vi "HEWH RLT PRAT.vi"() -> ()   [LabVIEW 2016] (continued)
      n10 = local write "Outlet Valve A"(w132) -> ()
      n11 = local write "Outlet Valve B"(w132) -> ()
      n12 = local write "Outlet Valve C"(w132) -> ()
      n13 = local write "Outlet Valve D"(w132) -> ()
      n14 = local write "Draw Complete"(w135) -> ()
      n15 = local write "DAQ Finished"(w135) -> ()
      n16 = local write "Init Complete"(w134) -> ()
      n17 = local write "Finish"(w134) -> ()
      n18 = local write "Alarm A"(w134) -> ()
      n19 = local write "Alarm B"(w134) -> ()
      n20 = local write "Start Draw Loop"(w134) -> ()
      n21 = local write "Alarm C"(w134) -> ()
      n22 = local write "Start/Pause test"(w134) -> ()
      n23 = local write "Alarm D"(w134) -> ()
      n24 = local write "Use Agilent?"(w134) -> ()
      n25 = local write "Disable Station 1"(w137) -> ()
      n26 = local write "Disable Station 2"(w137) -> ()
      n27 = local write "Disable Station 3"(w137) -> ()
      n28 = local write "Disable Station 4"(w137) -> ()
      n29 = local write "Shutdown"("" ("Shutdown")) -> ()
      n30 = disable-structure shown="Disabled" {
        frame Disabled {
          n31 = call "UTILITY Startup and Initialize.vi"() -> ()  [unwired: 24 in, 4 out]
        }
        frame Enabled {
        }
      }
    }
  }
  n32 = call "HEWH Power Notifier.vi"("Status"=w99, "error in (no error)"=w105, "Set Status"=w98, "name (unnamed)"="PowerA") -> ("error out"=w104:errorcluster)  [unwired: 6 in, 1 out]
  n33 = call "HEWH Power Notifier.vi"("Status"=w99, "error in (no error)"=w104, "Set Status"=w98, "name (unnamed)"="PowerB") -> ("error out"=w102:errorcluster)  [unwired: 6 in, 1 out]
  n34 = call "HEWH Power Notifier.vi"("Status"=w99, "error in (no error)"=w102, "Set Status"=w98, "name (unnamed)"="PowerC") -> ("error out"=w101:errorcluster)  [unwired: 6 in, 1 out]
  n35 = call "HEWH Power Notifier.vi"("Status"=w99, "error in (no error)"=w101, "Set Status"=w98, "name (unnamed)"="PowerD") -> ("error out"=w55:errorcluster)  [unwired: 6 in, 1 out]
  n36 = Current VI's Path() -> (path=w58:path)
  n37 = call "UTILITY This VIs Path.vi"("path"=w58, "error in (no error)"=w55) -> ("Folder Path"=w53:path, "FileVersionInfo Out"=w59:T5, "error out"=w54:errorcluster)  [unwired: 7 in, 4 out]
  n38 = Unbundle By Name(w59) -> ("FileVersion"=→"File  Version":string)
  n39 = call "HEWH Read Settings.vi"("Tool Base Path"=w53, "Error In"=w54) -> ("K-Factor Intellifaucet"=→"K-Factor Intellifaucet":dbl, "Power Analyzer"=→"Power Analyzer":T11, "Station"=→"Station":string, "LV Program"=w64:T24, "Error Out"=w65:errorcluster)  [unwired: 13 in]
  "LV Program" <- w64
  n40 = case shown="\"HEWH\", Default" w64 {
    tunnel: [Save_File_RLT_Station_Type."Single Station" ("RLT Station Type") Save_File_RLT_Station_Type."Four Stations" ("RLT Station Type")] -> w52
    frame "HEWH", Default {
      w140 = FALSE ("New File Per CycA")
      n41 = local write "New File Per CycA"(w140) -> ()
      n42 = local write "New File Per CycB"(w140) -> ()
      n43 = local write "New File Per CycC"(w140) -> ()
      n44 = local write "New File Per CycD"(w140) -> ()
    }
    frame "PRAT", "HEWH RLT" {
      w142 = TRUE ("New File Per CycA")
      n45 = local write "New File Per CycA"(w142) -> ()
      n46 = local write "New File Per CycB"(w142) -> ()
      n47 = local write "New File Per CycC"(w142) -> ()
      n48 = local write "New File Per CycD"(w142) -> ()
    }
  }
  n49 = call <vilib>:"Obtain Semaphore Reference.vi"("error in (no error)"=w65, "name (unnamed)"="MW100") -> ("error out"=w96:errorcluster, "semaphore"=w78:T56)  [unwired: 3 in, 1 out]
  n50 = Create User Event(user event datatype=w110, error in=w96) -> (user event=w24:refnum<user-event>, error out=w108:errorcluster)
  n51 = Create User Event(user event datatype=w109, error in=w108) -> (user event=w107:refnum<user-event>, error out=w82:errorcluster)
  n52 = Create User Event(user event datatype=w83, error in=w82) -> (user event=w23:refnum<user-event>, error out=w1:errorcluster)
  n53 = Create User Event(user event datatype=w68, error in=w1) -> (user event=w67:refnum<user-event>, error out=w63:errorcluster)
  n54 = Obtain Queue(name (unnamed)="Start Draw", element data type=T54 {"Start Draw"=FALSE, "Station ID"=enum."A", "Station Draw Info"={"Sequence #"=0.0, "Cycles"=0, "Mode Setting"="", "Flow Rate (GPM)"=0.0, "Temperature (F)"=0.0, "Reset Timer"=FALSE, "Use Temp Decline Method"=FALSE, "Terminate Condition"=enum."C1-Terminate Draw @ Gallon Mark", "Condition Value #1"=0.0, "UE"=FALSE, "LE"=FALSE, "Comp"=FALSE, "Fan"=FALSE, "Test End Time (Sec)"=0.0, "Purge Until Cutout"=FALSE, "Start Conditions"=enum."Heat Source Cutout", "Condition Value #2"=0.0, "Remove Power"=FALSE, "Time"=0.0, "Check Special Cond."=enum."SC2-Check Heat Source (On-C2/Off-C1)", "Condition#"=enum."C1", "Draw Flags"=enum."N/A", "Data Processing Delay (FHD 15sec, UEF 5 Sec)"=0.0, "Test Complete"=FALSE}, "Send Condition"=enum."N/A"}, error in (no error)=w63) -> (queue out=w116:refnum<queue>, error out=w3:errorcluster)  [unwired: 2 in, 1 out]
  n55 = call "UTILITY String Notifier.vi"("Status"=UTILITY_Notifier."Set", "error in (no error)"=w3, "Set Status"="", "name (unnamed)"="TimerA") -> ("error out"=w6:errorcluster)  [unwired: 6 in, 1 out]
  n56 = call "UTILITY String Notifier.vi"("Status"=UTILITY_Notifier."Set", "error in (no error)"=w6, "Set Status"="", "name (unnamed)"="TimerB") -> ("error out"=w5:errorcluster)  [unwired: 6 in, 1 out]
  n57 = call "UTILITY String Notifier.vi"("Status"=UTILITY_Notifier."Set", "error in (no error)"=w5, "Set Status"="", "name (unnamed)"="TimerC") -> ("error out"=w4:errorcluster)  [unwired: 6 in, 1 out]
  n58 = call "UTILITY String Notifier.vi"("Status"=UTILITY_Notifier."Set", "error in (no error)"=w4, "Set Status"="", "name (unnamed)"="TimerD") -> ("error out"=w2:errorcluster)  [unwired: 6 in, 1 out]
  n59 = call "UTILITY String Notifier.vi"("Status"=UTILITY_Notifier."Set", "error in (no error)"=w2, "Set Status"="", "name (unnamed)"="Message") -> ("error out"=w92:errorcluster)  [unwired: 6 in, 1 out]
  n60 = register-events(w107, w23) -> (reference out=w86:refnum<event-registration>)  [unwired: 2 in, 1 out]
  n61 = call "UTILITY Boolean Notifier.vi"("Status"=UTILITY_Notifier."Set", "error in (no error)"=w92, "Set Status"=FALSE, "name (unnamed)"="Stop Custom Draw") -> ("error out"=w74:errorcluster)  [unwired: 6 in, 1 out]
  n62 = call "HEWH Draw Flag.vi"("Station ID"=Station_ID_Selector."Global", "Status"=UTILITY_Notifier."Set", "Error In"=w74) -> ("Error Out"=w73:errorcluster)  [unwired: 8 in, 4 out]
  n63 = Bundle By Name(cluster="File Locations In", "General Setup Paths.Tool Base Path"=w53) -> (w56:T2)
  n64 = call "HEWH Cut Out Flag.vi"("Error In"=w73) -> ("Error Out"=w69:errorcluster)  [unwired: 10 in]
  n65 = call "UTILITY Boolean Notifier.vi"("Status"=UTILITY_Notifier."Set", "error in (no error)"=w69, "Set Status"=FALSE, "name (unnamed)"="Use Last Start Condition") -> ("error out"=w29:errorcluster)  [unwired: 6 in, 1 out]
  n66 = call "HEWH GEA Notifier.vi"("Status"=UTILITY_Notifier."Set", "error in (no error)"=w29, "name (unnamed)"="GEA_A") -> ("error out"=w28:errorcluster)  [unwired: 7 in, 1 out]
  n67 = call "HEWH GEA Notifier.vi"("Status"=UTILITY_Notifier."Set", "error in (no error)"=w28, "name (unnamed)"="GEA_B") -> ("error out"=w27:errorcluster)  [unwired: 7 in, 1 out]
  n68 = call "HEWH GEA Notifier.vi"("Status"=UTILITY_Notifier."Set", "error in (no error)"=w27, "name (unnamed)"="GEA_C") -> ("error out"=w26:errorcluster)  [unwired: 7 in, 1 out]
  n69 = call "HEWH GEA Notifier.vi"("Status"=UTILITY_Notifier."Set", "error in (no error)"=w26, "name (unnamed)"="GEA_D") -> ("error out"=w25:errorcluster)  [unwired: 7 in, 1 out]
  n70 = case shown="\"Single Station\", Default" w52 {
    tunnel: [w145 w156] -> w50
    tunnel: [w145 w155] -> w49
    tunnel: [w145 w154] -> w48
    tunnel: [w146 w153] -> w46
    tunnel: [w146 w152] -> w62
    tunnel: [w146 w151] -> w61
    tunnel: w56 -> [_ w150]
    tunnel: [w144 w149] -> w21
    tunnel: [w144 w148] -> w20
    tunnel: [w144 w147] -> w19
    frame "Single Station", Default {
      w144 = T2 {"General Setup Paths"={"Calibration File Path"=path "", "DOE Capacity Path"=path "", "Data Folder Path"=path "", "RLT Backup Data Path"=path "", "Tool Base Path"=path "", "General Startup Config Path"=path "", "File Save Previous Run Path"=path "", "File Save Configuration Data Path"=path ""}, "Data File Paths"={"Data File Path"=path "", "Debug File Path"=path "", "Bus Log Path"=path "", "Current"=path "", "Summary"=path ""}, "New Summary Created"=FALSE, "Check Location Interval (Second)"=0} ("File Locations Out")
      w145 = T28 {"Appliance Details"={"FileVersionInfo"={"FileVersion"="", "ProductName"="", "InternalName"="", "CompanyName"="", "LegalCopyright"="", "FileDescription"=""}, "Dishwasher Info"={"Open Cup Weight (gm):"=0.0, "Auto Cup Weight (gm):"=0.0, "Detergent-Dish:"="", "Inlet Temperature-Dish:"="", "Cycle Mode-Dish:"="", "Unit Control-Dish:"="", "Manufacturer-Dish:"=""}, "Washer Info"={"Hot Water Temperature (Fahrenheit):"="", "Cold Water Temperature (Fahrenheit):"="", "Capacity (cu.ft):"=0.0, "Initial Cloth Weight:"=0.0, "Cloth Lot:"=0, "Model Family:"="", "Program Name:"="", "Cycle Selection:"="", "Wash Temperature:"="", "Rinse Temperature:"="", "Load Size:"=""}, "File Name Output Array"=[], "Calibration Output Array"=[], "Appliance Common"={"Engineer:"="", "Model Number:"="", "Serial Number:"="", "Comments:"="", "Station ID:"="", "Technician:"="", "TR Number:"="", "Lab ID:"="", "Voltage:"="", "Water Pressure (PSI):"="", "Test Date:"="", "Computer Name:"="", "IP Address:"="", "Ambient RH:"="", "Frequency:"="", "Build:"="", "Filename:"="", "Test Type:"="", "Load Run #:"=0, "Ambient Temperature (F):"="", "File Path:"=path "", "Cycles Per Year"=60}, "Water Heater"={"Heating Mode:"=""}, "Dryer"={"Heat Setting:"="", "Washer Water Temperature (60 ± 5°F):"=60, "Water Hardness (PPM):"=17, "Dryness Setting:"="", "Dryer Type:"="", "Exhaust:"="", "Drying Cycle:"="", "Load Type:"="", "Nominal Load Weight"="", "Dryer Initial IMC Data"={"Measured IMC (lbs)"=7.0, "Actual Initial RMC (%)"=7.0, "RMC (Desired %)"=100.0, "Bone Dry Wt(lbs)"=7.0, "Tolerance(%)"=5.0, "Actual Final RMC (%)"=0.0, "CEF (lbf/kWh)"=0.0, "Minimum Weight (lbf)"=0.0, "Average Weight (lbf)"=0.0, "Maximum Weight (lbf)"=0.0, "Measured IMC In Range?"=FALSE, "Moisture Reduction Factor"=55.5, "Field Use Factor"=1.04, "Empty Dryer Cold Weigth"=0.0, "Energy Standard"=enum."D2-Automatic Dryer", "Weight Cloth (lbs)"=0.0, "Relative Moisture Content (%)"=0.0, "Relative Moisture Content - Avg (%)"=0.0}}}, "Display Data (RLT)"={"Status Color"=0, "Serial Number Display"="", "Cycle Count Display"=0, "Station Label Display"="", "Current Run Start Time Display"=0.0, "Board ID Display"="", "RPM Display"=0, "Current Display"=0.0, "Current Path Display"=path "", "Saving Display"=FALSE, "Unit Type Display"=enum."", "Total Time On Display"=0.0, "UI Button"=FALSE}} ("Main Washer Display Out")
      w146 = T57 {"GEA Diagnostic Data - Washer"={"Speed (RPM)"=0, "Load Size"=0, "Temperature"=0, "Water Pressure"=0.0, "Detergent"=0, "Fabric Softener"=0, "Tub Direction"="", "Detergent Valve"=FALSE, "Fabric Softener Valve"=FALSE, "Recirculating Pump"=FALSE, "Drain Valve"=FALSE, "Hot Valve"=FALSE, "Cold Valve"=FALSE, "Lid Closed Status"="", "Lid Lock Status"="", "Error Count"=0, "IGBT Temperature (Deg C)"=0, "Motor Speed"=0, "Latched OOB"=0, "Raw OOB"=0, "Plaster Status"=0, "Inverter Power (W)"=0, "Target Speed(BRPM)"=0, "Latched Agitate Motor Temp (Deg C)"=0, "Current Motor Temp (Deg C)"=0, "Profiler Status"="", "Current Inverter Action"="", "Error Codes"="", "Lid Locked"=FALSE, "Lid Closed"=FALSE, "9E Diagnostic Data"={"Total Cycle Time (Min)"=0, "Total Cycle Count (Current)"=0, "Total Error Count"=0, "Machine Error History"=0, "Washer UI History"=0, "Inverter Error History"=0, "Cycle Storage Limit"=0, "Error Storage Limit"=0, "Cycle Pages Supported"=0, "Error Pages Supported"=0, "Inverter Reset Count"=0}, "9F Diagnostic Data"={"Cycle Buffer Index"="", "Page Number"="", "Total Cycle Count"=0, "Delay Start Time"=0, "Stain Selected"="", "Selected Cycle"=0, "eWash"="", "Soil Level"="", "Temperature"="", "Overnight Ready"="", "Spin Setting"="", "Control Lock Status"="", "Stain Remover"="", "Steam Assist"="", "My Cycle"="", "PreWash"="", "Debug Log Enabled"="", "Rinse"="", "Signal Level"="", "PreSoak"=""}}, "Software Version"={"Critical Major SW Version"="", "Critical Minor SW Version"="", "Major SW Version"="", "Minor SW Version"="", "Parametric Data Ver. Major"="", "Parametric Data Ver. Minor"="", "Diagnostics Data Ver. Major"="", "Diagnostics Data Ver. Minor"="", "Current Personality Setting"=""}, "Debug Search Parameters"={"Pause"=["MchStdby", "MchPz", "MchIdl", "Machine Standby", "Machine Pause", "Machine Idle"], "Run"=["MchRn", "Machine Run", "Resume Process"], "EOC"=["EOC"], "Error Codes"=["Error1", "try", "rty", "inverr"]}, "Message Count"=0, "Number of Messages"=0, "Partial Message String"="", "Full Message to Save"="", "Board ID"="", "Board Index"=0, "Source Address"=0, "Destination Address"=0, "Data to send"=[], "ReceivedData"=[], "Debug/GEA Data"=[], "Command"=0, "GEA2 Reference Out"=refnum, "GEA2 Event Registration"=refnum, "Bus Data"="", "GEA Data"=[], "Network Variable Location"=0, "Water Heater GEA2 Data"={"GEA2 Label Array"=[], "PID_PARAMETERS"=[], "SUPPORTED_MODES"=[], "Button Status"={"Switch 1"=FALSE, "Switch 2"=FALSE, "Switch 3"=FALSE, "Switch 4"=FALSE, "Switch 5"=FALSE, "Switch 6"=FALSE, "Switch 7"=FALSE, "Switch 8"=FALSE, "Switch 9"=FALSE, "Switch 10"=FALSE, "Switch 11"=FALSE, "Switch 12"=FALSE, "Switch 13"=FALSE, "Switch 14"=FALSE, "Switch 15"=FALSE, "Switch 16"=FALSE}, "Status Query"={"Days Remaining (For Std Electric and Vacation)"=0, "Unit Status"="", "Current Tank Temp in Deg F"=0, "Current Setpoint in Deg F"=0, "Filter Status (% used)"=0, "Fallback Status (Fallback heating mode)"="", "Fallback Temp"=0, "\"Set Mode\" Selection"=""}, "Service Error Codes"={"Reserved"=FALSE, "Reserved 1"=FALSE, "Reserved 2"=FALSE, "Reserved 3"=FALSE, "Reserved 4"=FALSE, "Reserved 5"=FALSE, "Reserved 6"=FALSE, "Reserved 7"=FALSE, "DataFlash Fail Status"=FALSE, "Stuck Key Fail Status"=FALSE, "Dry Tank Fail Status"=FALSE, "Miswire Fail Status"=FALSE, "Reserved 8"=FALSE, "Reserved 9"=FALSE, "Reserved 10"=FALSE, "Reserved 11"=FALSE, "UE Fail Status"=FALSE, "LE Fail Status"=FALSE, "Filter Fail Status"=FALSE, "T3A Fail Status"=FALSE, "T3B Fail Status"=FALSE, "T4 Fail Status"=FALSE, "T5 Fail Status"=FALSE, "T2 Fail Status"=FALSE, "SS Cond A Status"=FALSE, "SS Cond B Status"=FALSE, "SS Cond C Status"=FALSE, "SS Cond D Status"=FALSE, "SS Cond E Status"=FALSE, "SS Cond F Status"=FALSE, "SS Fan Status"=FALSE, "CMP Fail Status"=FALSE}, "HEM_KWH_DATA"=[], "OTHER_FAULT_COUNTS"=[], "GEA2 Raw Message"="", "Hyperterminal Data"={"Source"=0, "Destination"=0, "Command"=0, "Length"=0, "CRC"=0, "UE - state (1/0 on off)"=0, "LE - state (1/0 on off)"=0, "Comp - state (1/0 on off)"=0, "Fan  - state (1/0 on off)"=0, "Setpoint Deg F"=0, "T2(TankSensor)"=0.0, "T3A(EvapIn)"=0.0, "T3B(EvapOut)"=0.0, "T4(CompressorDischarge)"=0.0, "T5(Ambient)"=0.0, "Current"=0.0, "Voltage (Volts)"=0, "EEV Position (0-480)"=0, "Reason for last heating cycle termination"=0, "Reason Data word 1"="", "Reason Data word 2"="", "Reason Data word 3"="", "Reason Data word 4"="", "SW Debug Data"="", "Flow Events (Bit Encoded)"=0, "Heating Control Mode"=0}, "Extra Data"={"Water Capacity (Gallons)"=0, "Max Vacation Duration Days"=0, "Min Vacation Duration Days"=0, "Max Set Point (Deg F)"=0, "Min Set Point (Deg F)"=0, "T5 Resistance"=0, "T4 Resistance"=0, "T3B Resistance"=0, "T2 Resistance"=0, "STD_ELEC_RANGE"="", "SS_FAULT_COUNTS"="", "SERIAL_NUMBER"="", "READ_PERSONALITY"=0, "RQST_OVERRIDE_STATUS"="", "MODEL_SELECT_AD_VALUE"=0, "MODEL NUMBER"="", "IDLB_RESISTANCE"=0, "DSM Override Status"="", "RQST_DATA_FROM_Memory"="", "RQST_DATA_FROM_DATA_FLASH"="", "RQST_CURRENT_PID_SH_TARGET"=0, "Unit System Mode"=""}}} ("GEA Information Out")
    }
    frame "Four Stations" {
      n71 = call "UTILITY Read Config File Start BUS.vi"("Station ID"="StationB", "File Locations In"=w150) -> ("Main Washer Display Out"=w156:T28, "GEA Information Out"=w153:T57, "File Locations Out"=w149:T2)  [unwired: 6 in, 1 out]
      n72 = call "UTILITY Read Config File Start BUS.vi"("Station ID"="StationC", "File Locations In"=w150) -> ("Main Washer Display Out"=w155:T28, "GEA Information Out"=w152:T57, "File Locations Out"=w148:T2)  [unwired: 6 in, 1 out]
      n73 = call "UTILITY Read Config File Start BUS.vi"("Station ID"="StationD", "File Locations In"=w150) -> ("Main Washer Display Out"=w154:T28, "GEA Information Out"=w151:T57, "File Locations Out"=w147:T2)  [unwired: 6 in, 1 out]
    }
  }
  n74 = case shown="\"HEWH\", Default" w64 {
    tunnel: ["Data: Initialize\nInitialize Equipment\nGet Software Version A\nUpdate File Locations\nLoad Configuration\nInit Hot Laurel" "Data: Initialize\nInitialize Equipment\nGet Software Version A\nGet Software Version B\nGet Software Version C\nGet Software Version D\nUpdate File Locations\nLoad Configuration"] -> w124
    frame "HEWH", Default {
    }
    frame "PRAT", "HEWH RLT" {
    }
  }
  n75 = call "UTILITY Read Config File Start BUS.vi"("Station ID"="StationA", "File Locations In"=w56) -> ("Main Washer Display Out"=w51:T28, "GEA Information Out"=w47:T57, "File Locations Out"=w22:T2)  [unwired: 6 in, 1 out]
  n76 = register-events(w24, w67) -> (reference out=w84:refnum<event-registration>)  [unwired: 2 in, 1 out]
  n77 = call <vilib>:"Add State(s) to Queue__jki_lib_state_machine.vi"("State(s) in (\"\")"="Data: Initialize\nMain Power") -> ("States Out"=w126:string)  [unwired: 14 in]
  n78 = call <vilib>:"Add State(s) to Queue__jki_lib_state_machine.vi"("State(s) in (\"\")"=w124) -> ("States Out"=w123:string)  [unwired: 14 in]
  n79 = while {
    tunnel: w25 -> [w162]
    tunnel: [w162] -> w81
    stop <- w163 stop-if-true
    n80 = local read "Start Draw Loop"() -> (w163:bool)
    n81 = Wait Until Next ms Multiple(millisecond multiple=u32 250) -> ()  [unwired: 1 out]
  }
  n82 = call <vilib>:"Add State(s) to Queue__jki_lib_state_machine.vi"("State(s) in (\"\")"=w127) -> ("States Out"=w130:string)  [unwired: 14 in]
  n83 = while {
    i -> [w183]
    stop <- w184 stop-if-true
    w178 = UTILITY_Notifier."Read" ("Status")
    n84 = call "UTILITY String Notifier.vi"("Status"=w178, "name (unnamed)"="Message") -> ("error out"=w182:errorcluster, "latest notification"=w170:string)  [unwired: 8 in]
    "Message" <- w170
    n85 = local read "Disable Station 1"() -> (w168:T31)
    n86 = call "UTILITY String Notifier.vi"("Status"=w178, "error in (no error)"=w182, "name (unnamed)"="MessageA") -> ("error out"=w181:errorcluster, "latest notification"=w173:string)  [unwired: 7 in]
    n87 = case shown="\"Enable Station\"" w168 {
      tunnel: w173 -> [_ w202]
      tunnel: w170 -> [_ w200]
      frame "Disable Station (No Draw)", Default {
      }
      frame "Enable Station" {
        n88 = call "HEWH Message Filter.vi"("Main Display?"=TRUE, "Station Message"=w202, "Main Message"=w200) -> ("Combined Message"=→"Message A" →"Message A Detail":string)  [unwired: 7 in, 1 out]
      }
    }
    n89 = local read "Disable Station 2"() -> (w167:T31)
    n90 = call "UTILITY String Notifier.vi"("Status"=w178, "error in (no error)"=w181, "name (unnamed)"="MessageB") -> ("error out"=w180:errorcluster, "latest notification"=w172:string)  [unwired: 7 in]
    n91 = case shown="\"Disable Station (No Draw)\", Default" w167 {
      tunnel: w172 -> [_ w198]
      tunnel: w170 -> [_ w196]
      frame "Disable Station (No Draw)", Default {
      }
      frame "Enable Station" {
        n92 = call "HEWH Message Filter.vi"("Main Display?"=TRUE, "Station Message"=w198, "Main Message"=w196) -> ("Combined Message"=→"Message B" →"Message B Detail":string)  [unwired: 7 in, 1 out]
      }
    }
    n93 = local read "Disable Station 3"() -> (w166:T31)
    n94 = call "UTILITY String Notifier.vi"("Status"=w178, "error in (no error)"=w180, "name (unnamed)"="MessageC") -> ("error out"=w179:errorcluster, "latest notification"=w171:string)  [unwired: 7 in]
    n95 = case shown="\"Disable Station (No Draw)\", Default" w166 {
      tunnel: w171 -> [_ w194]
      tunnel: w170 -> [_ w192]
      frame "Disable Station (No Draw)", Default {
      }
      frame "Enable Station" {
        n96 = call "HEWH Message Filter.vi"("Main Display?"=TRUE, "Station Message"=w194, "Main Message"=w192) -> ("Combined Message"=→"Message C" →"Message C Detail":string)  [unwired: 7 in, 1 out]
      }
    }
    n97 = local read "Disable Station 4"() -> (w165:T31)
    n98 = call "UTILITY String Notifier.vi"("Status"=w178, "error in (no error)"=w179, "name (unnamed)"="MessageD") -> ("latest notification"=w169:string)  [unwired: 7 in, 1 out]
    n99 = case shown="\"Disable Station (No Draw)\", Default" w165 {
      tunnel: w170 -> [_ w190]
      tunnel: w169 -> [_ w189]
      frame "Disable Station (No Draw)", Default {
      }
      frame "Enable Station" {
        n100 = call "HEWH Message Filter.vi"("Main Display?"=TRUE, "Station Message"=w189, "Main Message"=w190) -> ("Combined Message"=→"Message D" →"Message D Detail":string)  [unwired: 7 in, 1 out]
      }
    }
    n101 = local read "DAQ Finished"() -> (w184:bool)
    n102 = Wait Until Next ms Multiple(millisecond multiple=u32 500) -> ()  [unwired: 1 out]
    "Read Message Loop" <- w183
  }
  n103 = while "Main Test Process Loop" {
    shift-right: [w225] -> _
    shift-left: _ -> [w224]
    shift-right: [w227] -> w117
    shift-left: w25 -> [w222]
    shift-right: [w226] -> _
    shift-left: w130 -> [w228]
    tunnel: [w221] -> w128
    shift-right: [w220] -> _
    shift-left: string[] [] -> [w219]
    tunnel: w78 -> [w216]
    tunnel: w116 -> [w215]
    tunnel: [w214] -> w118
    tunnel: w84 -> [w212]
    tunnel: w47 -> [w210]
    tunnel: w46 -> [w209]
    tunnel: w62 -> [w208]
    tunnel: w61 -> [w207]
    tunnel: w51 -> [w206]
    tunnel: w50 -> [w205]
    tunnel: w49 -> [w204]
    tunnel: w48 -> [w203]
    i -> [w211]
    stop <- w221 stop-if-true
    # "Main Test Process Loop"
    n104 = call <vilib>:"Parse State Queue__JKI_lib_State_Machine.vi"("State Queue"=w228, "Error In (no error)"=w222) -> ("Remaining States"=w229:string, "Current State"=w217:string, "Arguments"=w218:string)  [unwired: 11 in]
    "Main State" <- w217
    n105 = case shown="\"Test: Wait for Power Off (Station B)\"" w217 {
      selector: w217 -> [_ _ w446 _ _ _ _ _ _ _ _ _ _ _ _ _ _ _ _ _ _ _ _ _ _ _ _ _ _ _ _ _ _ _ _ _ _ _ _]
      tunnel: w229 -> [w242 w444 w450 w469 w501 w511 w542 w563 w567 w576 w581 w586 w608 w613 w621 w693 w705 w736 w742 w753 w758 w792 w812 w826 w840 w854 w902 w972 w1042 w1112 w1140 w1146 w1159 w1169 w1179 w1189 w1202 w1281 w1319]
      tunnel: w218 -> [_ _ _ _ _ _ _ _ _ _ _ _ _ _ _ w688 w699 _ _ _ _ _ _ _ _ _ _ _ _ _ _ _ _ _ _ _ w1197 _ _]
      tunnel: w224 -> [w240 w441 w448 w460 w499 w508 w528 w561 w568 w573 w578 _ w606 w610 w619 w691 w701 w733 w739 w750 w755 w788 w809 w823 w837 w851 w899 w969 w1039 w1109 w1135 w1148 w1156 w1166 w1176 w1186 w1194 w1279 w1311]
      tunnel: [w239 w442 w452 w466 w490 w506 w533 w543 errorcluster {"status"=FALSE, "code"=0, "source"=""} ("error out") w572 w579 w584 w602 w611 w618 w689 w702 w734 w740 w751 w756 w759 w806 w820 w834 w848 w875 w944 w1014 w1084 w1141 w1147 w1150 w1160 w1170 w1180 w1199 w1278 w1315] -> w227
      tunnel: w222 -> [w238 w442 w451 w466 w495 w506 w530 w544 w565 w572 w579 w584 w604 w611 w618 w690 w703 w734 w740 w751 w756 w779 w806 w820 w834 w848 w855 w925 w995 w1065 w1141 w1147 w1152 w1162 w1172 w1182 w1196 w1278 w1301]
      tunnel: [w241 w443 w449 w468 w500 w510 w541 w562 w570 w575 w580 w585 w607 w612 w620 w692 w704 w735 w741 w752 w757 w791 w811 w825 w839 w853 w901 w971 w1041 w1111 w1142 w1149 w1158 w1168 w1178 w1188 w1201 w1280 w1318] -> w226
      tunnel: [_ _ _ _ _ _ _ _ _ TRUE _ _ _ _ _ _ _ _ _ _ _ _ _ _ _ _ _ _ _ _ _ _ _ _ _ _ _ _ _] -> w221
      tunnel: [w237 w441 w448 w467 w475 w507 w527 w561 w568 w573 w578 w583 w606 w610 w619 w691 w701 w733 w739 w750 w755 w790 w807 w821 w835 w849 w898 w968 w1038 w1108 w1135 w1148 w1156 w1166 w1176 w1186 w1194 w1279 w1311] -> w225
      tunnel: 250 ("Timeout") -> [w236 _ _ _ _ _ _ _ _ _ _ _ _ _ _ _ _ _ _ _ _ _ _ _ _ _ _ _ _ _ _ _ _ _ _ _ _ _ _]
      tunnel: w216 -> [_ _ _ _ _ _ _ _ _ _ _ _ _ _ _ _ _ _ _ _ _ _ _ _ _ _ _ _ _ _ _ _ _ _ _ _ _ _ _]
      tunnel: w215 -> [w235 w440 w445 w457 w477 w509 w536 w560 w564 w571 w577 w582 w603 w609 w616 w687 w698 w732 w737 w743 w754 w789 w810 w824 w838 w852 w900 w970 w1040 w1110 w1136 w1145 w1157 w1167 w1177 w1187 w1200 w1277 w1314]
      tunnel: [w235 w440 w445 w457 w477 w509 w536 w560 w564 w571 w577 w582 w603 w609 w616 w687 w698 w732 w737 w743 w754 w789 w810 w824 w838 w852 w900 w970 w1040 w1110 w1136 w1145 w1157 w1167 w1177 w1187 w1200 w1277 w1312] -> w214
      tunnel: w212 -> [w234 _ _ _ _ _ _ _ _ _ _ _ _ _ _ _ _ _ _ _ _ _ _ _ _ _ _ _ _ _ _ _ _ _ _ _ _ _ _]
      tunnel: w210 -> [_ _ _ _ _ _ _ _ _ _ _ _ _ _ _ _ _ _ _ _ _ _ _ _ _ _ _ _ _ _ _ _ _ _ _ _ w1193 _ _]
      tunnel: w209 -> [_ _ _ _ _ _ _ _ _ _ _ _ _ _ _ _ _ _ _ _ _ _ _ _ _ _ _ _ _ _ _ _ _ _ _ _ w1192 _ _]
      tunnel: w208 -> [_ _ _ _ _ _ _ _ _ _ _ _ _ _ _ _ _ _ _ _ _ _ _ _ _ _ _ _ _ _ _ _ _ _ _ _ w1191 _ _]
      tunnel: w207 -> [_ _ _ _ _ _ _ _ _ _ _ _ _ _ _ _ _ _ _ _ _ _ _ _ _ _ _ _ _ _ _ _ _ _ _ _ w1190 _ _]
      tunnel: w206 -> [_ _ _ _ _ w505 _ _ _ _ _ _ _ _ _ _ _ _ _ _ _ _ _ _ _ _ _ _ _ _ _ _ _ _ _ _ _ _ _]
      tunnel: w205 -> [_ _ _ _ _ w504 _ _ _ _ _ _ _ _ _ _ _ _ _ _ _ _ _ _ _ _ _ _ _ _ _ _ _ _ _ _ _ _ _]
      tunnel: w204 -> [_ _ _ _ _ w503 _ _ _ _ _ _ _ _ _ _ _ _ _ _ _ _ _ _ _ _ _ _ _ _ _ _ _ _ _ _ _ _ _]
      tunnel: w203 -> [_ _ _ _ _ w502 _ _ _ _ _ _ _ _ _ _ _ _ _ _ _ _ _ _ _ _ _ _ _ _ _ _ _ _ _ _ _ _ _]
      frame "", "Idle" {
        n106 = event shown="[0] Timeout" {
          selector: w234 -> [_ _ _ _ _ _]
          dyn-events: _ -> [_ _ _ _ _ _]
          timeout: w236 -> [_ _ _ _ _ _]
          tunnel: w242 -> [w250 w318 w328 w342 w387 w422]
          tunnel: [w251 w317 w327 w342 w387 w422] -> w241
          tunnel: w240 -> [w246 w315 w329 w344 w386 w425]
          tunnel: [w245 w316 w319 w348 w381 w420] -> w239
          tunnel: w238 -> [w248 w316 w320 w348 w383 w421]
          tunnel: [w246 w315 w329 w343 w385 w423] -> w237
          event Timeout {
            n107 = event-data() -> ()  [unwired: 1 in, 1 out]
            n108 = local read "LV Program"() -> (w244:T24)
            n109 = case shown="\"HEWH\", Default" w244 {
              tunnel: ["Test: Update Display A\nCheck for UI Event" "Test: Update Display A\nTest: Update Display B\nTest: Update Display C\nTest: Update Display D\nCheck for UI Event"] -> w247
              frame "HEWH", Default {
              }
              frame "PRAT", "HEWH RLT" {
              }
            }
            n110 = case shown="True" "Start/Pause test" {
              tunnel: [w257 w265] -> w249
              tunnel: w248 -> [w254 w269]
              tunnel: [w256 w268] -> w245
              tunnel: w247 -> [w257 w267]
              tunnel: w246 -> [_ w264]
              frame False {
                n111 = local read "Start Draw Loop"() -> (w255:bool)
                n112 = case shown="True" w255 {
                  tunnel: w254 -> [w258 w260]
                  tunnel: [w258 w259] -> w256
                  frame False {
                  }
                  frame True {
                    n113 = call "UTILITY String Notifier.vi"("Status"=UTILITY_Notifier."Set", "error in (no error)"=w260, "Set Status"=T7 "Select Test Sequence to Enable Start Button...." ("Message"), "name (unnamed)"="Message") -> ("error out"=w259:errorcluster)  [unwired: 6 in, 1 out]
                  }
                }
              }
              frame True {
                n114 = First Call?() -> (First Call?: T/F=w270:bool)
                n115 = case shown="True" w270 {
                  tunnel: w269 -> [w277 w309]
                  tunnel: [w273 w308] -> w268
                  tunnel: w264 -> [w276 _]
                  frame False {
                    n116 = while {
                      tunnel: w276 -> [w293]
                      shift-right: [w288] -> w274
                      shift-left: w277 -> [w294]
                      shift-right: [w284] -> _
                      shift-left: _ -> [w283]
                      stop <- TRUE stop-if-true
                      n117 = Increment(x=w283) -> (x+1=w284:dbl)
                      n118 = Unbundle By Name(w293) -> ("Station A Display.Display Data (RLT)"=w292:T29, "Station B Display.Display Data (RLT)"=w291:T29, "Station C Display.Display Data (RLT)"=w290:T29, "Station D Display.Display Data (RLT)"=w289:T29)
                      n119 = local read "Test CompleteD"() -> (w278:bool)
                      n120 = local read "Test CompleteC"() -> (w279:bool)
                      n121 = local read "Test CompleteB"() -> (w280:bool)
                      n122 = local read "Test CompleteA"() -> (w281:bool)
                      n123 = Quotient & Remainder(x=w284, y=4) -> (x-y*floor(x/y)=w285:i32)  [unwired: 1 out]
                      n124 = Equal To 0?(x=w285) -> (x = 0?=w282:bool)
                      "Update Heating Message" <- w282
                      n125 = case shown="True" w282 {
                        tunnel: w294 -> [w295 w305]
                        tunnel: w292 -> [_ w304]
                        tunnel: w291 -> [_ w303]
                        tunnel: w290 -> [_ w302]
                        tunnel: w289 -> [_ w301]
                        tunnel: [w295 w300] -> w288
                        tunnel: w281 -> [_ w299]
                        tunnel: w280 -> [_ w298]
                        tunnel: w279 -> [_ w297]
                        tunnel: w278 -> [_ w296]
                        frame False {
                        }
                        frame True {
                          n126 = call "HEWH Update Message.vi"("Display Data (RLT) A"=w304, "Test CompleteA"=w299, "Test CompleteB"=w298, "Test CompleteC"=w297, "Test CompleteD"=w296, "Display Data (RLT) B"=w303, "Display Data (RLT) C"=w302, "Display Data (RLT) D"=w301, "error in (no error)"=w305) -> ("error out"=w300:errorcluster)  [unwired: 6 in]
                        }
                      }
                    }
                    n127 = call "UTILITY String Notifier.vi"("Status"=UTILITY_Notifier."Set", "error in (no error)"=w274, "Set Status"="", "name (unnamed)"="Message") -> ("error out"=w273:errorcluster)  [unwired: 6 in, 1 out]
                  }
                  frame True {
                    w306 = FALSE ("Show Stand Override Flow Data A")
                    w307 = TRUE ("Reset Timer")
                    n128 = local write "Reset Timer (Main)"(w307) -> ()
                    n129 = local write "Reset Timer (A)"(w307) -> ()
                    n130 = local write "Reset Timer (B)"(w307) -> ()
                    n131 = local write "Reset Timer (C)"(w307) -> ()
                    n132 = local write "Reset Timer (D)"(w307) -> ()
                    n133 = local write "Show Stand Override Flow Data A"(w306) -> ()
                    n134 = local write "Show Stand Override Flow Data B"(w306) -> ()
                    n135 = local write "Show Stand Override Flow Data C"(w306) -> ()
                    n136 = local write "Show Stand Override Flow Data D"(w306) -> ()
                    n137 = call "UTILITY String Notifier.vi"("Status"=UTILITY_Notifier."Set", "error in (no error)"=w309, "Set Status"=T7 "Starting Test...." ("Message"), "name (unnamed)"="Message") -> ("error out"=w308:errorcluster)  [unwired: 6 in, 1 out]
                  }
                }
                n138 = call <vilib>:"Add State(s) to Queue__jki_lib_state_machine.vi"("State(s) in Front (\"\")"="Test: Check Complete", "State(s) in (\"\")"=w267) -> ("States Out"=w265:string)  [unwired: 13 in]
              }
            }
            n139 = call <vilib>:"Add State(s) to Queue__jki_lib_state_machine.vi"("State(s) in Front (\"\")"=w249, "State(s) in (\"\")"=w250) -> ("States Out"=w251:string)  [unwired: 13 in]
          }
          event Panel Close? {
            n140 = event-data() -> ()  [unwired: 1 in, 1 out]
            n141 = call <vilib>:"Add State(s) to Queue__jki_lib_state_machine.vi"("State(s) in Front (\"\")"="Macro: Exit", "State(s) in (\"\")"=w318) -> ("States Out"=w317:string)  [unwired: 13 in]
            n142 = event-data("Discard?"=TRUE) -> ()  [unwired: 1 in, 1 out]
          }
          event Menu Selection (User) {
            n143 = event-data() -> ("ItemTag"=w323:string)  [unwired: 1 in, 6 out]
            n144 = call <vilib>:"Trim Whitespace.vi"("string"=w323) -> ("trimmed string"=w325:string)  [unwired: 1 in]
            n145 = call <vilib>:"Trim Whitespace.vi"("string"="Exit") -> ("trimmed string"=w326:string)  [unwired: 1 in]
            n146 = Equal?(x=w325, y=w326) -> (x = y?=w322:bool)
            n147 = case shown="False" w322 {
              tunnel: ["" "Macro: Exit"] -> w321
              tunnel: w320 -> [w330 w333]
              tunnel: [w330 w332] -> w319
              frame False {
              }
              frame True {
                n148 = for {
                  N: 10 -> [_]
                  shift-right: [w337] -> w332
                  shift-left: w333 -> [w338]
                  n149 = call "UTILITY Boolean Notifier.vi"("Status"=UTILITY_Notifier."Set", "error in (no error)"=w338, "Set Status"=TRUE, "name (unnamed)"="Stop Custom Draw") -> ("error out"=w337:errorcluster)  [unwired: 6 in, 1 out]
                  n150 = Wait Until Next ms Multiple(millisecond multiple=u32 10) -> ()  [unwired: 1 out]
                }
              }
            }
            n151 = call <vilib>:"Add State(s) to Queue__jki_lib_state_machine.vi"("State(s) in Front (\"\")"=w321, "State(s) in (\"\")"=w328) -> ("States Out"=w327:string)  [unwired: 13 in]
          }
          event User Event {
            n152 = event-data() -> ()  [unwired: 1 in, 5 out]
            n153 = local read "Station ID to Reset"() -> (w345:T25)
            n154 = local read "Updated Cycle Count"() -> (w347:i32)
            n155 = local read "Reset Cycle Count"() -> (w346:bool)
            n156 = case shown="\"A\", Default" w345 {
              tunnel: [w352 w360 w367 w375] -> w343
              tunnel: w346 -> [w351 w359 w368 w376]
              tunnel: w347 -> [w350 w358 w366 w374]
              tunnel: w344 -> [w349 w357 w365 w373]
              frame "A", Default {
                n157 = case shown="True" w351 {
                  tunnel: w349 -> [w353 w356]
                  tunnel: [w353 w355] -> w352
                  tunnel: w350 -> [_ w354]
                  frame False {
                  }
                  frame True {
                    n158 = Bundle By Name(cluster=w356, "Station A Display.Display Data (RLT).Cycle Count Display"=w354) -> (w355:T70)
                  }
                }
              }
              frame "B" {
                n159 = case shown="True" w359 {
                  tunnel: w357 -> [w361 w364]
                  tunnel: [w361 w363] -> w360
                  tunnel: w358 -> [_ w362]
                  frame False {
                  }
                  frame True {
                    n160 = Bundle By Name(cluster=w364, "Station B Display.Display Data (RLT).Cycle Count Display"=w362) -> (w363:T70)
                  }
                }
              }
              frame "C" {
                n161 = case shown="True" w368 {
                  tunnel: w365 -> [w369 w372]
                  tunnel: [w369 w371] -> w367
                  tunnel: w366 -> [_ w370]
                  frame False {
                  }
                  frame True {
                    n162 = Bundle By Name(cluster=w372, "Station C Display.Display Data (RLT).Cycle Count Display"=w370) -> (w371:T70)
                  }
                }
              }
              frame "D" {
                n163 = case shown="False" w376 {
                  tunnel: w373 -> [w377 w380]
                  tunnel: [w377 w379] -> w375
                  tunnel: w374 -> [_ w378]
                  frame False {
                  }
                  frame True {
                    n164 = Bundle By Name(cluster=w380, "Station D Display.Display Data (RLT).Cycle Count Display"=w378) -> (w379:T70)
                  }
                }
              }
            }
          }
          event User Event {
            n165 = event-data() -> ()  [unwired: 1 in, 5 out]
            n166 = local read "Draw Station"() -> (w384:string)
            n167 = case shown="\"A\"" w384 {
              tunnel: w386 -> [w391 w395 w402 w408 w416]
              tunnel: [w391 w394 w401 w407 w415] -> w385
              tunnel: w383 -> [w390 w392 w399 w406 w413]
              tunnel: [w390 w392 w399 w406 w413] -> w382
              frame Default {
              }
              frame "A" {
                n168 = Unbundle By Name(w395) -> ("Station A Display.Display Data (RLT)"=w398:T29)
                n169 = call "PRAT Update Status Color.vi"("Disable Cycle Counter"=FALSE, "Draw Station is Drawing Water"=TRUE, "Display Data (RLT) In"=w398) -> ("Display Data (RLT) Out"=w396:T29)  [unwired: 7 in, 1 out]
                n170 = Bundle By Name(cluster=w395, "Station A Display.Display Data (RLT)"=w396) -> (w394:T70)
              }
              frame "B" {
                n171 = Unbundle By Name(w402) -> ("Station B Display.Display Data (RLT)"=w405:T29)
                n172 = call "PRAT Update Status Color.vi"("Disable Cycle Counter"=FALSE, "Draw Station is Drawing Water"=TRUE, "Display Data (RLT) In"=w405) -> ("Display Data (RLT) Out"=w403:T29)  [unwired: 7 in, 1 out]
                n173 = Bundle By Name(cluster=w402, "Station B Display.Display Data (RLT)"=w403) -> (w401:T70)
              }
              frame "C" {
                n174 = Unbundle By Name(w408) -> ("Station C Display.Display Data (RLT)"=w411:T29)
                n175 = call "PRAT Update Status Color.vi"("Disable Cycle Counter"=FALSE, "Draw Station is Drawing Water"=TRUE, "Display Data (RLT) In"=w411) -> ("Display Data (RLT) Out"=w409:T29)  [unwired: 7 in, 1 out]
                n176 = Bundle By Name(cluster=w408, "Station C Display.Display Data (RLT)"=w409) -> (w407:T70)
              }
              frame "D" {
                n177 = Unbundle By Name(w416) -> ("Station D Display.Display Data (RLT)"=w419:T29)
                n178 = call "PRAT Update Status Color.vi"("Disable Cycle Counter"=FALSE, "Draw Station is Drawing Water"=TRUE, "Display Data (RLT) In"=w419) -> ("Display Data (RLT) Out"=w417:T29)  [unwired: 7 in, 1 out]
                n179 = Bundle By Name(cluster=w416, "Station D Display.Display Data (RLT)"=w417) -> (w415:T70)
              }
            }
            n180 = flat-sequence {
              tunnel: w382 -> [w388]
              tunnel: [w388] -> w381
              frame #0 {
                n181 = local write "Draw Station"("") -> ()
              }
            }
          }
          event "Start/Pause test": Value Change {
            n182 = event-data() -> ("NewVal"=w424:bool)  [unwired: 1 in, 5 out]
            n183 = case shown="False" w424 {
              tunnel: w425 -> [w431 w439]
              tunnel: [w429 w439] -> w423
              tunnel: w421 -> [w427 w438]
              tunnel: [w426 w438] -> w420
              frame False {
                n184 = global read "Save File Globals HCC.vi" "Startup"() -> (w430:u32)
                n185 = Bundle By Name(cluster=w431, "Station A Display.Display Data (RLT).Status Color"=w430, "Station B Display.Display Data (RLT).Status Color"=w430, "Station C Display.Display Data (RLT).Status Color"=w430, "Station D Display.Display Data (RLT).Status Color"=w430) -> (w429:T70)
                n186 = for {
                  N: 10 -> [_]
                  shift-right: [w433] -> w426
                  shift-left: w427 -> [w434]
                  n187 = call "UTILITY Boolean Notifier.vi"("Status"=UTILITY_Notifier."Set", "error in (no error)"=w434, "Set Status"=TRUE, "name (unnamed)"="Stop Custom Draw") -> ("error out"=w433:errorcluster)  [unwired: 6 in, 1 out]
                  n188 = Wait Until Next ms Multiple(millisecond multiple=u32 10) -> ()  [unwired: 1 out]
                }
              }
              frame True {
              }
            }
          }
        }
      }
      frame "---------- Core ----------" {
        n189 = call <vilib>:"Add State(s) to Queue__jki_lib_state_machine.vi"("State(s) in (\"\")"=w444) -> ("States Out"=w443:string)  [unwired: 14 in]
      }
      frame Default {
        w455 = 42 items=["No error", "Argument error", "Memory is full", "Out of zone", "End of file", "File already open", "Generic file I/O error", "File not found", "File permission error", "Disk is full", "Duplicate path", "Too many files open", "System feature not enabled", "Resource file not found", "Cannot add resource", "Resource not found", "Image not found", "Image memory error", "Pen does not exist", "Config type invalid", "Config token not found", "Config parse error", "Config memory error", "Bad external code format", "Bad external code offset", "External code not present", "Null window", "Destroy window error", "Null menu", "Print aborted", "Bad print record", "Print driver error", "Windows error during printing", "Memory error during printing", "Print dialog error", "Generic print error", "Invalid device refnum", "Device not found", "Device parameter error", "Device unit error", "Cannot open device", "Device call aborted", "Generic error", "Cancelled by user", "Object ID too low", "Object ID too high", "Object not in heap", "Unknown heap", "Unknown object (invalid DefProc)", "Unknown object (DefProc not in table)", "Message out of range", "Invalid (null) method", "Unknown message", "Manager call not supported", "Bad address", "Network operation in progress", "Network operation timed out", "Connection is busy", "Network attribute not supported", "Network error", "Address in use", "System out of memory", "Connection aborted", "Connection refused", "Not connected", "Already connected", "Connection closed", "Initialization error (interapplication manager)", "Bad occurrence", "Wait on unbound occurrence handler", "Occurrence queue overflow", "Datalog type conflict", "Unused", "Unrecognized type (interapplication manager)", "Memory corrupt", "Failed to make temporary DLL", "Old CIN version", "Drag socket not found", "Failed to load drop-object", "Failed to register OLE object", "Failed to release OLE object", "Format specifier type mismatch", "Unknown format specifier", "Too few format specifiers", "Too many format specifiers", "Scan failed", "Newer CIN version", "Error converting to variant", "Runtime menu error", "Password tampered", "Variant attribute not found", "Incompatible variant data type", "Event data is not available", "Event Store is not present", "Occurrence is not found", "Event Queue is not created", "Event info is not available", "Refnum passed is NULL", "Error retrieving Class GUID", "Error retrieving CoClass GUID", "Error retrieving TypeLib GUID.", "Bad built application magic bytes.", "Specific driver is different from the specific driver associated with the Logical Name.", "There is no session opened to the class driver.", "Max Error", "MAX - Error with config objects", "MAX - Error loading configuration", "MAX - Group not supported"]
        # "Current State"
        # "Handle mistyped state name (developer tool)"
        n190 = Format Into String(format string="Software Exception: Unhandled State \"%s\"." ("message"), error in=w451, w446) -> (resulting string=w454:string, error out=w453:errorcluster)  [unwired: 1 in]
        n191 = call <vilib>:"Error Cluster From Error Code.vi"("show call chain? (False)"=TRUE, "error in (no error)"=w453, "error message (\"\")"=w454, "error code (0)"=w455) -> ("error out"=w452:errorcluster)  [unwired: 5 in]
        n192 = call <vilib>:"Add State(s) to Queue__jki_lib_state_machine.vi"("State(s) in (\"\")"=w450) -> ("States Out"=w449:string)  [unwired: 14 in]
      }
      frame "Initialize Core Data" {
        # "If panel starts closed or is an EXE, then close it when we exit"
        n193 = property class="App"() -> ("App.Kind"=w464:T65)  [unwired: 2 in, 2 out]
        n194 = control-ref of="Current VI Reference"() -> (w458:refnum<vi>)
        n195 = property class="VI"() -> ("Front Panel.Open"=w465:bool)  [unwired: 2 in, 2 out]
        n196 = Not(x=w465) -> (.not. x?=w462:bool)
        n197 = Equal?(x=w464, y=T65."Run Time System" ("Application:Kind")) -> (x = y?=w461:bool)
        n198 = Or(x=w462, y=w461) -> (x .or. y?=w459:bool)
        n199 = Bundle By Name(cluster=w460, "Core.Current VI Reference"=w458, "Core.Close Panel on Exit?"=w459) -> (w467:T70)
        n200 = call <vilib>:"Add State(s) to Queue__jki_lib_state_machine.vi"("State(s) in (\"\")"=w469) -> ("States Out"=w468:string)  [unwired: 14 in]
      }
      frame "Initialize Channels" {
        w486 = T71 0 items=["both", "start of string", "end of string"] ("location (both)")
        # "The channel list is compiled here"
        n201 = local read "LV Program"() -> (w476:T24)
        n202 = call "HEWH RLT Channel Test Labels.vi"("LV Program"=w476, "Error In"=w495) -> ("Station A"=w494:T72, "Station B"=w493:T72, "Station C"=w492:T72, "Station D"=w491:T72, "Error Out"=w490:errorcluster)  [unwired: 9 in]
        n203 = call "HEWH RLT Label Parse.vi"("Station A"=w494) -> ("Agilent Channel List"=w481:string[][], "MW100 Channel List"=w482:string[][])  [unwired: 6 in, 3 out]
        n204 = call "HEWH RLT Label Parse.vi"("Station A"=w493) -> ("Agilent Channel List"=w479:string[][], "MW100 Channel List"=w480:string[][])  [unwired: 6 in, 3 out]
        n205 = call "HEWH RLT Label Parse.vi"("Station A"=w492) -> ("Agilent Channel List"=w484:string[][], "MW100 Channel List"=w485:string[][])  [unwired: 6 in, 3 out]
        n206 = call "HEWH RLT Label Parse.vi"("Station A"=w491) -> ("Agilent Channel List"=w483:string[][], "MW100 Channel List"=w478:string[][])  [unwired: 6 in, 3 out]
        n207 = Build Array (concatenate)(w481, w479, w484, w483) -> (w488:string[][])
        n208 = Index Array(array=w488, index (col)=1 ("disabled index (col)")) -> (element=w487:string[])  [unwired: 1 in]
        n209 = Array To Spreadsheet String(delimiter (Tab)="," ("format string"), array=w487, 3:"%s" ("format string")) -> (spreadsheet string=w496:string)
        n210 = call <vilib>:"Trim Whitespace.vi"("string"=w496, "location (both)"=w486) -> ("trimmed string"=w473:string)
        "Analog Channel-List" <- w473
        n211 = Bundle By Name(cluster=w499, "RLT Station Channels.MW100.Station A Channels, MW100"=w482, "RLT Station Channels.Agilent.Station A Channels, Agilent"=w481, "RLT Station Channels.MW100.Station B Channels, MW100"=w480, "RLT Station Channels.Agilent.Station B Channels, Agilent"=w479, "RLT Station Channels.Agilent.Station C Channels, Agilent"=w484, "RLT Station Channels.MW100.Station C Channels, MW100"=w485, "RLT Station Channels.Agilent.Station D Channels, Agilent"=w483, "RLT Station Channels.MW100.Station D Channels, MW100"=w478) -> (w475:T70)
        n212 = call <vilib>:"Add State(s) to Queue__jki_lib_state_machine.vi"("State(s) in (\"\")"=w501) -> ("States Out"=w500:string)  [unwired: 14 in]
        n213 = Equal?(x=w473, y="") -> (x = y?=w471:bool)
        n214 = Not(x=w471) -> (.not. x?=→"Use Agilent?":bool)
        n215 = Unbundle By Name(w475) -> ("RLT Station Channels"=w474:T46)
        n216 = local write "RLT Station Channels"(w474) -> ()
      }
      frame "Initialize Files" {
        n217 = Bundle By Name(cluster=w508, "Station A Display"=w505, "Station B Display"=w504, "Station C Display"=w503, "Station D Display"=w502) -> (w507:T70)
        n218 = call <vilib>:"Add State(s) to Queue__jki_lib_state_machine.vi"("State(s) in (\"\")"=w511) -> ("States Out"=w510:string)  [unwired: 14 in]
      }
      frame "Init Complete" {
        n219 = Unbundle By Name(w528) -> ("Station A Display.Display Data (RLT)"=w529:T29, "Station B Display.Display Data (RLT)"=w522:T29, "Station C Display.Display Data (RLT)"=w521:T29, "Station D Display.Display Data (RLT)"=w520:T29)
        n220 = call "PRAT Update Status Color.vi"("Disable Cycle Counter"=TRUE, "Disable Station"=HEWH_RLT_Station_Disable."Disable Station (No Draw)", "Display Data (RLT) In"=w529) -> ("Display Data (RLT) Out"=w518:T29)  [unwired: 7 in, 1 out]
        n221 = call "PRAT Update Status Color.vi"("Disable Cycle Counter"=TRUE, "Disable Station"=HEWH_RLT_Station_Disable."Disable Station (No Draw)", "Display Data (RLT) In"=w522) -> ("Display Data (RLT) Out"=w517:T29)  [unwired: 7 in, 1 out]
        n222 = call "PRAT Update Status Color.vi"("Disable Cycle Counter"=TRUE, "Disable Station"=HEWH_RLT_Station_Disable."Disable Station (No Draw)", "Display Data (RLT) In"=w521) -> ("Display Data (RLT) Out"=w516:T29)  [unwired: 7 in, 1 out]
        n223 = call "PRAT Update Status Color.vi"("Disable Cycle Counter"=TRUE, "Disable Station"=HEWH_RLT_Station_Disable."Disable Station (No Draw)", "Display Data (RLT) In"=w520) -> ("Display Data (RLT) Out"=w515:T29)  [unwired: 7 in, 1 out]
        n224 = call <vilib>:"Add State(s) to Queue__jki_lib_state_machine.vi"("State(s) in (\"\")"=w542) -> ("States Out"=w541:string)  [unwired: 14 in]
        n225 = call "UTILITY String Notifier.vi"("Status"=UTILITY_Notifier."Set", "error in (no error)"=w530, "Set Status"="", "name (unnamed)"="Draw Station") -> ("error out"=w532:errorcluster)  [unwired: 6 in, 1 out]
        n226 = Bundle By Name(cluster=w528, "Station A Display.Display Data (RLT)"=w518, "Station B Display.Display Data (RLT)"=w517, "Station C Display.Display Data (RLT)"=w516, "Station D Display.Display Data (RLT)"=w515) -> (w527:T70)
        n227 = call "UTILITY String Notifier.vi"("Status"=UTILITY_Notifier."Set", "error in (no error)"=w532, "Set Status"=T7 "Initializing Complete...." ("Message"), "name (unnamed)"="Message") -> ("error out"=w533:errorcluster)  [unwired: 6 in, 1 out]
        "Init Complete" <- TRUE ("Init Complete")
      }
      frame "Save Status" {
        n228 = Unbundle By Name(w561) -> ("Station A Display"=w559:T28, "Station B Display"=w556:T28, "Station C Display"=w546:T28, "Station D Display"=w545:T28)
        n229 = local read "File Locations A"() -> (w558:T2)
        n230 = call "HCC Read Write Display.vi"("Read Write Control"=enum16{"Read", "Write"}."Write", "error in (no error)"=w544, "Washer Input"=w559, "File Locations In"=w558) -> ("error out"=w553:errorcluster)  [unwired: 6 in, 1 out]
        n231 = local read "File Locations B"() -> (w555:T2)
        n232 = call "HCC Read Write Display.vi"("Read Write Control"=enum16{"Read", "Write"}."Write", "error in (no error)"=w553, "Washer Input"=w556, "File Locations In"=w555) -> ("error out"=w550:errorcluster)  [unwired: 6 in, 1 out]
        n233 = local read "File Locations C"() -> (w552:T2)
        n234 = call "HCC Read Write Display.vi"("Read Write Control"=enum16{"Read", "Write"}."Write", "error in (no error)"=w550, "Washer Input"=w546, "File Locations In"=w552) -> ("error out"=w547:errorcluster)  [unwired: 6 in, 1 out]
        n235 = local read "File Locations D"() -> (w549:T2)
        n236 = call "HCC Read Write Display.vi"("Read Write Control"=enum16{"Read", "Write"}."Write", "error in (no error)"=w547, "Washer Input"=w545, "File Locations In"=w549) -> ("error out"=w543:errorcluster)  [unwired: 6 in, 1 out]
        n237 = call <vilib>:"Add State(s) to Queue__jki_lib_state_machine.vi"("State(s) in (\"\")"=w563) -> ("States Out"=w562:string)  [unwired: 14 in]
      }
      frame "Error Handler" {
        # "Unhandled Error -- Display it"
        n238 = call <vilib>:"General Error Handler.vi"("error in (no error)"=w565) -> ()  [unwired: 10 in, 5 out]
        n239 = call <vilib>:"Add State(s) to Queue__jki_lib_state_machine.vi"("State(s) in Front (\"\")"="/* Post Error States", "State(s) in (\"\")"=w567) -> ("States Out"=w570:string)  [unwired: 13 in]
      }
      frame "Exit" {
        n240 = call <vilib>:"Add State(s) to Queue__jki_lib_state_machine.vi"("State(s) in (\"\")"=w576) -> ("States Out"=w575:string)  [unwired: 14 in]
      }
      frame "---------- Data ----------" {
        n241 = call <vilib>:"Add State(s) to Queue__jki_lib_state_machine.vi"("State(s) in (\"\")"=w581) -> ("States Out"=w580:string)  [unwired: 14 in]
      }
      frame "Data: Initialize" {
        n242 = flat-sequence {
          tunnel: [w597] -> w583
          frame #0 {
          }
          frame #1 {
            w588 = HEWH_Special_Condition_Check."N/A"  # Current Cond D
            w589 = HEWH_Special_Condition_Check."N/A"  # Current Cond C
            w590 = HEWH_Special_Condition_Check."N/A"  # Current Cond B
            w591 = HEWH_Special_Condition_Check."N/A"  # Current Cond A
            w599 = errorcluster[] []  # Error Log
            w600 = i32[] []  # DrawsLeft
            n243 = local read "Power Analyzer"() -> (w587:T11)
